vi "Initialize Filter State.vi"(9 "init (F)":bool, 10 "Filter State in":T2, 11 "IIR Filter Cluster":T1) -> (2 "Filter State out":T2, 3 "IIR Filter Cluster":T1)   [LabVIEW 2019, in "DSP.lvclass"]
uses:
  DSP.lvclass
  Typedefs/Filter State--Cluster.ctl
panel:
  out "reset?":bool
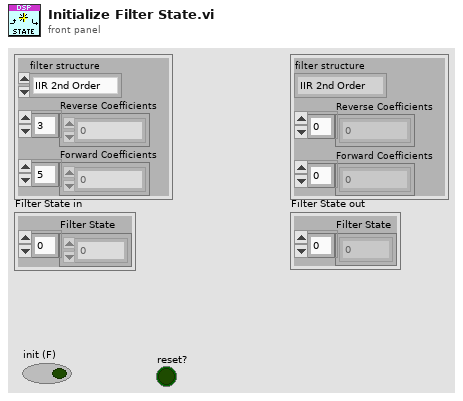
[diagram p1: front panel]
types:
  T1 = cluster{"filter structure":enum32{"IIR 2nd Order", "IIR 4th Order"}, "Reverse Coefficients":dbl[], "Forward Coefficients":dbl[]}
  T2 = typedef "DSP.lvclass/Filter State--Cluster.ctl" = cluster{"Filter State":dbl[]}
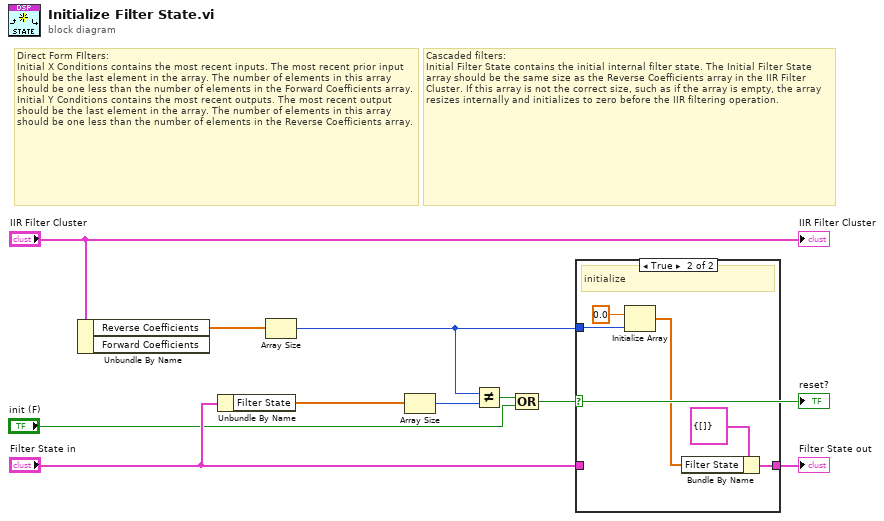
[diagram p0: block diagram]
diagram:
  # "Direct Form FIlters:\nInitial X Conditions contains the most recent inputs. The most recent prior input should be the last element in the array. The number of elements in this array should be one less than the number of elements in the Forward Coefficients array.  \nInitial Y Conditions contains the most recent outputs. The most recent output should be the last element in the array. The number of elements in this array should be one less than the number of elements in the Reverse Coefficients array."
  # "Cascaded filters:\nInitial Filter State contains the initial internal filter state. The Initial Filter State array should be the same size as the Reverse Coefficients array in the IIR Filter Cluster. If this array is not the correct size, such as if the array is empty, the array resizes internally and initializes to zero before the IIR filtering operation."
  n1 = Unbundle By Name("IIR Filter Cluster") -> ("Reverse Coefficients"=w9:dbl[])  [unwired: 1 out]
  n2 = Unbundle By Name("Filter State in") -> ("Filter State"=w5:dbl[])
  n3 = Array Size(array=w9) -> (size(s)=w1:i32)
  n4 = Array Size(array=w5) -> (size(s)=w6:i32)
  n5 = Not Equal?(x=w1, y=w6) -> (x != y?=w4:bool)
  n6 = Compound Arithmetic op=OR(w4, "init (F)") -> (w7:bool)
  "reset?" <- w7
  n7 = case shown="True" w7 {
    tunnel: "Filter State in" -> [w11 _]
    tunnel: [w11 w14] -> w3
    tunnel: w1 -> [_ w13]
    frame False {
    }
    frame True {
      # "initialize"
      n8 = Initialize Array(0.0 ("x"), w13) -> (w12:dbl[])
      n9 = Bundle By Name(cluster=T2 {"Filter State"=[]} ("s? t:f"), "Filter State"=w12) -> (w14:T2)
    }
  }
  "Filter State out" <- w3
  "IIR Filter Cluster" <- "IIR Filter Cluster"
